vi "autonSample.vi"(0 "Auton Array":dbl[][](array[numeric]), 5 "MeasuredHeading":dbl, 9 "EncoderDistance":dbl) -> (4 "Left Drive":dbl(knob) scale=-1.0..1.0, 6 "Right Drive":dbl(knob) scale=-1.0..1.0, 10 "Turret Rotation":dbl, 14 "Feeder motor":dbl, 15 "Shooter motor output":dbl)   [LabVIEW 2011]
uses:
  Robot Global Data.vi
panel:
  in  "ShooterDesRate 2":dbl
  in  "ShooterEncRate 2":dbl
  in  "ShooterDesRate":dbl
  in  "ShooterEncRate":dbl
  in  "Balls Fired 2":i32
  in  "Balls Fired":i32
  out "Tzero":i64
  out "AccumDist":dbl
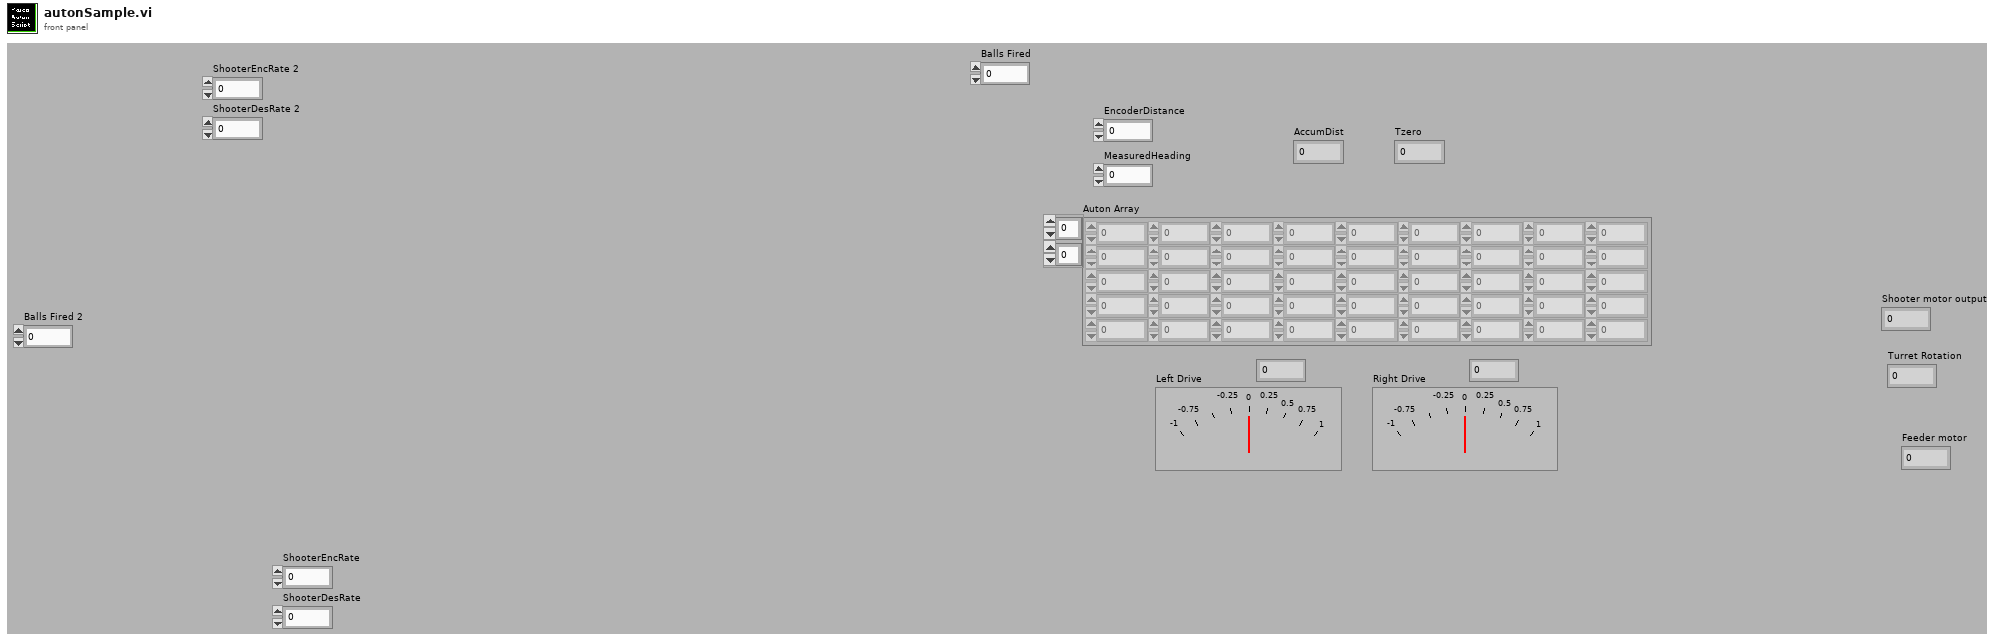
[diagram p1: front panel]
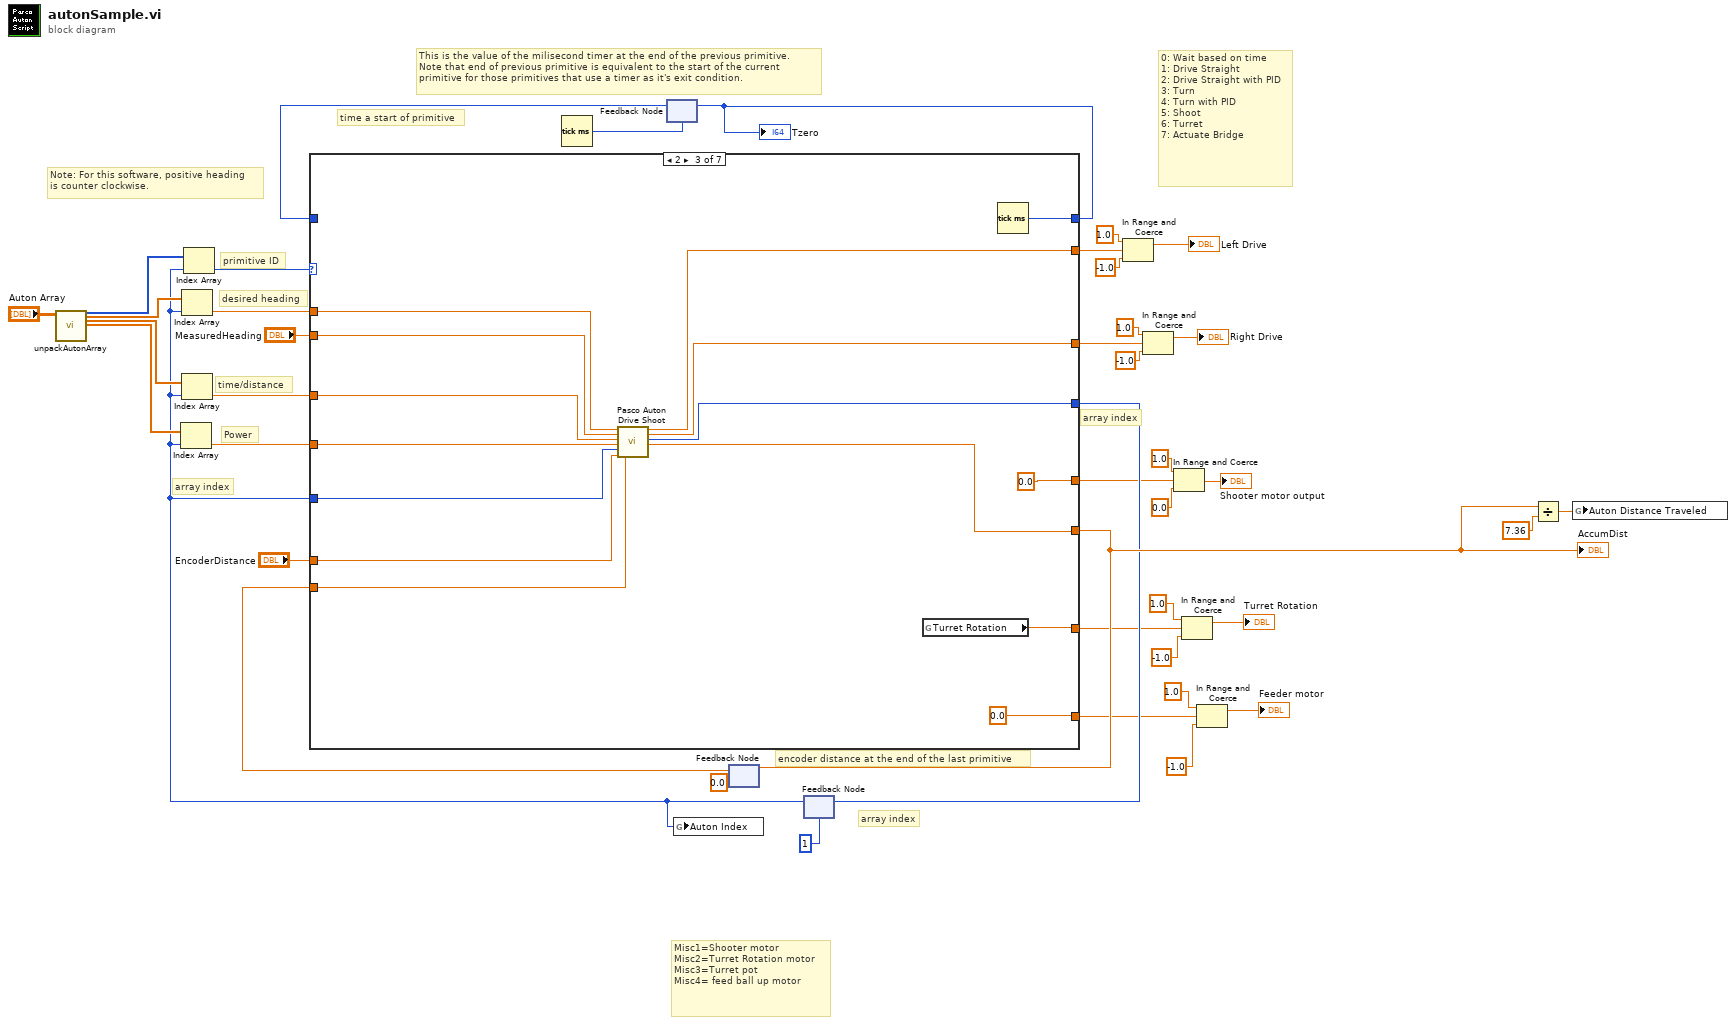
[diagram p0: block diagram]
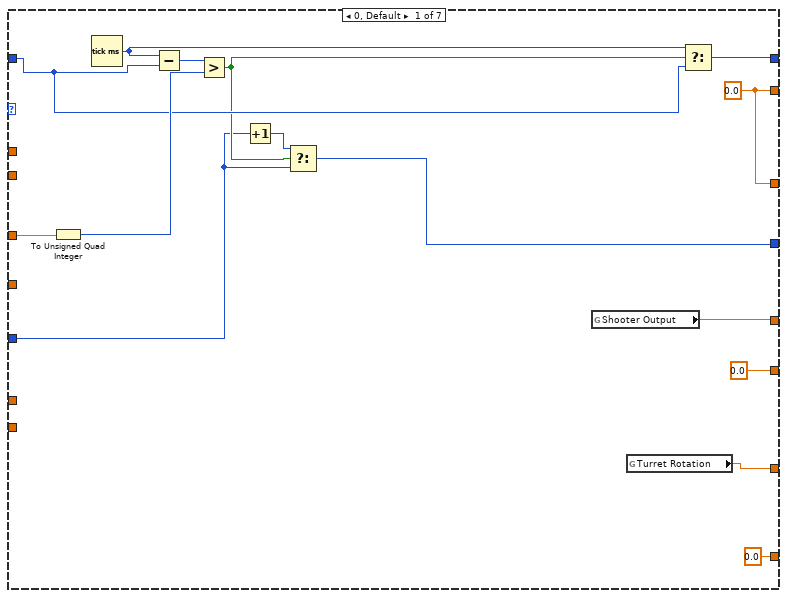
[diagram p2: hidden frame]
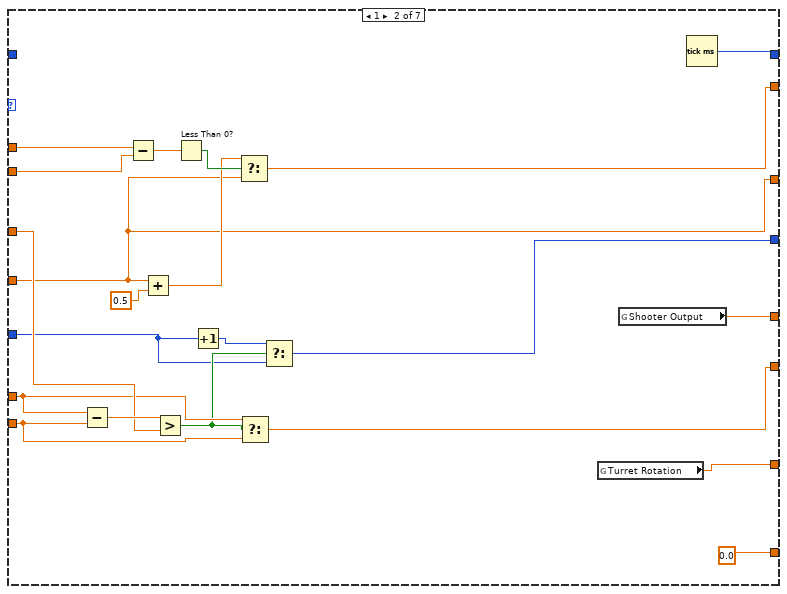
[diagram p3: hidden frame]
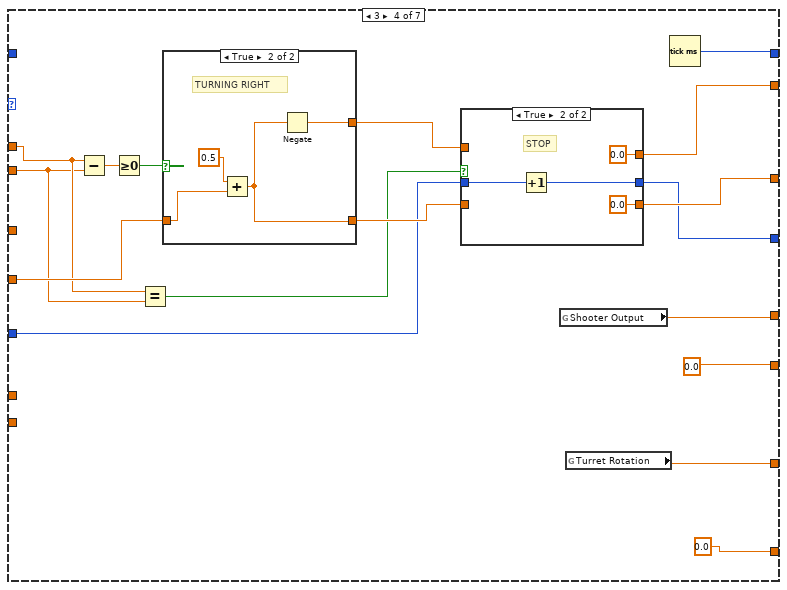
[diagram p4: hidden frame]
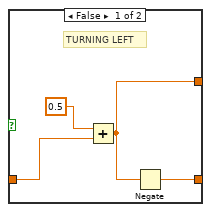
[diagram p6: hidden frame]
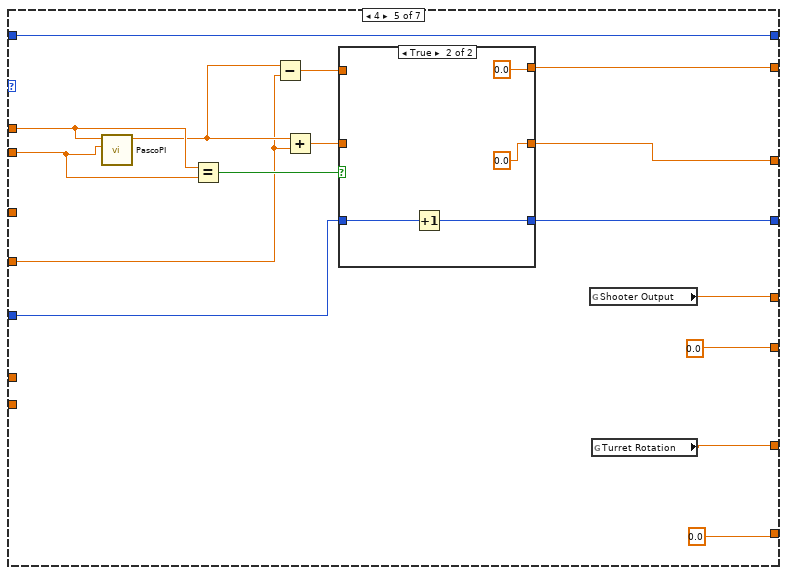
[diagram p7: hidden frame]
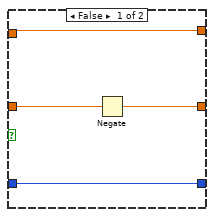
[diagram p8: hidden frame]
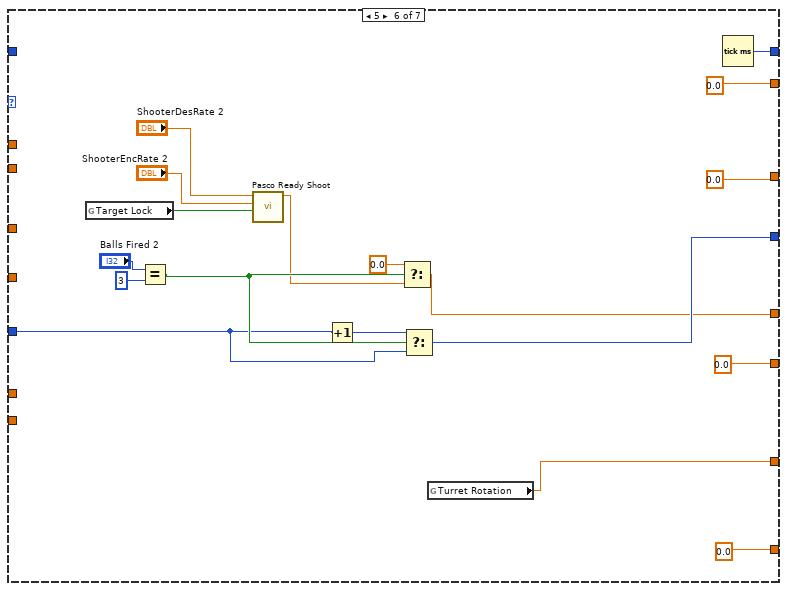
[diagram p9: hidden frame]
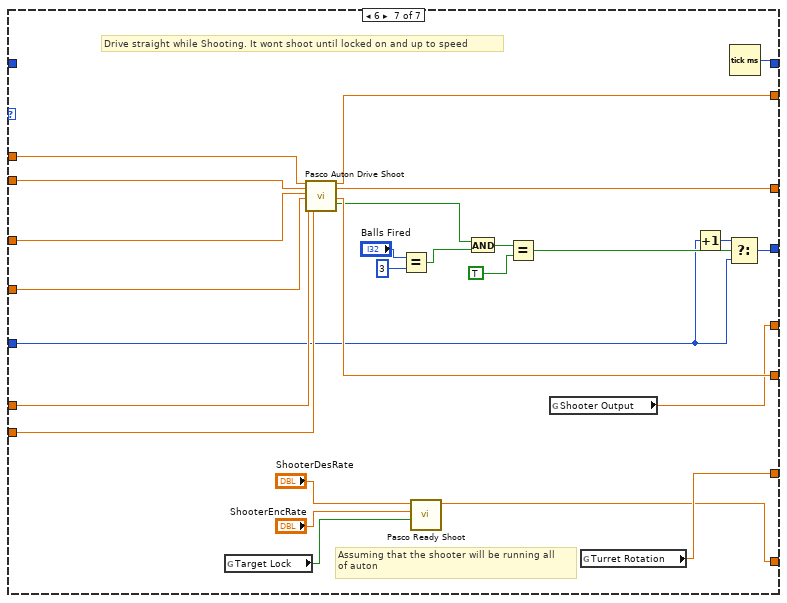
[diagram p10: hidden frame]
diagram:
  # "Misc1=Shooter motor\nMisc2=Turret Rotation motor\nMisc3=Turret pot\nMisc4= feed ball up motor"
  # "0: Wait based on time\n1: Drive Straight\n2: Drive Straight with PID\n3: Turn\n4: Turn with PID\n5: Shoot\n6: Turret\n7: Actuate Bridge"
  # "encoder distance at the end of the last primitive"
  # "Note: For this software, positive heading\nis counter clockwise."
  # "time a start of primitive"
  # "array index"
  # "array index"
  # "This is the value of the milisecond timer at the end of the previous primitive.\nNote that end of previous primitive is equivalent to the start of the current\nprimitive for those primitives that use a timer as it's exit condition."
  # "Power"
  # "array index"
  # "desired heading"
  # "primitive ID"
  # "time/distance"
  n1 = call "unpackAutonArray.vi"("all rows"="Auton Array") -> ("Primitive"=w41:i16[], "Heading"=w23:dbl[], "Distance/Time"=w24:dbl[], "Power"=w21:dbl[])  [unwired: 1 in, 22 out]
  n2 = Tick Count (ms)() -> (millisecond timer value=w35:u32)
  n3 = feedback #1(w35) -> (w39:u32)
  n4 = feedback #2(0.0 ("EncoderDistance")) -> (w20:dbl)
  n5 = feedback #3(1) -> (w2:i32)
  n6 = Index Array(array=w21, index=w2) -> (element=w37:dbl)
  n7 = Index Array(array=w23, index=w2) -> (element=w22:dbl)
  n8 = Index Array(array=w24, index=w2) -> (element=w38:dbl)
  n9 = Index Array(array=w41, index=w2) -> (element=w40:i16)
  n10 = case shown="2" w40 {
    tunnel: [w46 w63 w81 w99 w137 w161 w178] -> w15
    tunnel: w2 -> [w47 w64 w86 w98 w136 w154 w174]
    tunnel: [w57 w62 w92 w105 w141 w162 w172] -> w25
    tunnel: w39 -> [w53 _ _ _ w141 _ _]
    tunnel: w38 -> [w55 w71 w88 _ _ _ w191]
    tunnel: w22 -> [_ w77 w90 w107 w131 _ w193]
    tunnel: [w45 w73 w83 w101 w138 0.0 w187] -> w33
    tunnel: [w45 w59 w82 w104 w139 0.0 w186] -> w26
    tunnel: w37 -> [_ w59 w87 w109 w128 _ w190]
    tunnel: "EncoderDistance" -> [_ w70 w85 _ _ _ w189]
    tunnel: "MeasuredHeading" -> [_ w76 w89 w106 w132 _ w192]
    tunnel: [0.0 ("Encoder total") w67 w80 0.0 0.0 0.0 w185] -> w17
    tunnel: w20 -> [_ w69 w84 _ _ _ w188]
    tunnel: [w43 w58 0.0 ("Misc1  OUT") w94 w126 w160 w173] -> w11
    tunnel: [w44 w68 w79 w95 w127 w163 w176] -> w7
    tunnel: [0.0 ("Misc4 OUT") 0.0 0.0 0.0 0.0 0.0 w171] -> w3
    frame 0, Default {
      w45 = 0.0 ("Numeric")
      n11 = To Unsigned Quad Integer(1:w55) -> (0:w54:u64)
      n12 = Tick Count (ms)() -> (millisecond timer value=w52:u32)
      n13 = Subtract(x=w52, y=w53) -> (x-y=w56:u32)
      n14 = Greater?(x=w56, y=w54) -> (0:w49:bool)
      n15 = Increment(x=w47) -> (x+1=w48:i32)
      n16 = Select(t=w48, s=w49, f=w47) -> (s? t:f=w46:i32)
      n17 = global read "Robot Global Data.vi" "Shooter Output"() -> (w43:dbl)
      n18 = global read "Robot Global Data.vi" "Turret Rotation"() -> (w44:dbl)
      n19 = Select(t=w52, s=w49, f=w53) -> (s? t:f=w57:u32)
    }
    frame 1 {
      n20 = Subtract(x=w70, y=w69) -> (x-y=w72:dbl)
      n21 = Subtract(x=w77, y=w76) -> (x-y=w61:dbl)
      n22 = Add(x=w59, y=0.5) -> (x+y=w60:dbl)
      n23 = Greater?(x=w72, y=w71) -> (0:w66:bool)
      n24 = Less Than 0?(x=w61) -> (x < 0?=w75:bool)
      n25 = Increment(x=w64) -> (x+1=w65:i32)
      n26 = Select(t=w60, s=w75, f=w59) -> (s? t:f=w73:dbl)
      n27 = Select(t=w70, s=w66, f=w69) -> (s? t:f=w67:dbl)
      n28 = Select(t=w65, s=w66, f=w64) -> (s? t:f=w63:i32)
      n29 = global read "Robot Global Data.vi" "Turret Rotation"() -> (w68:dbl)
      n30 = global read "Robot Global Data.vi" "Shooter Output"() -> (w58:dbl)
      n31 = Tick Count (ms)() -> (millisecond timer value=w62:u32)
    }
    frame 2 {
      n32 = call "Pasco Auton Drive Shoot.vi"("Desired Heading"=w90, "Actual Heading"=w89, "time/distance"=w88, "Power"=w87, "Array"=w86, "Encoder total"=w85, "Encoder Return"=w84) -> ("Left Drive"=w83:dbl, "Right Drive"=w82:dbl, "Array Out"=w81:i32, "Encoder total"=w80:dbl)  [unwired: 8 in, 1 out]
      n33 = global read "Robot Global Data.vi" "Turret Rotation"() -> (w79:dbl)
      n34 = Tick Count (ms)() -> (millisecond timer value=w92:u32)
    }
    frame 3 {
      n35 = Subtract(x=w107, y=w106) -> (x-y=w110:dbl)
      n36 = Greater Or Equal To 0?(x=w110) -> (x >= 0?=w108:bool)
      n37 = Equal?(x=w107, y=w106) -> (x = y?=w100:bool)
      n38 = case shown="True" w108 {
        tunnel: w109 -> [w120 w122]
        tunnel: [w118 w124] -> w102
        tunnel: [w119 w123] -> w103
        frame False {
          # "TURNING LEFT"
          n39 = Add(x=0.5, y=w120) -> (x+y=w118:dbl)
          n40 = Negate(x=w118) -> (-x=w119:dbl)
        }
        frame True {
          # "TURNING RIGHT"
          n41 = Add(x=0.5, y=w122) -> (x+y=w123:dbl)
          n42 = Negate(x=w123) -> (-x=w124:dbl)
        }
      }
      n43 = case shown="True" w100 {
        tunnel: w98 -> [w113 w117]
        tunnel: [w113 w116] -> w99
        tunnel: [w112 0.0] -> w104
        tunnel: w103 -> [w112 _]
        tunnel: [w111 0.0] -> w101
        tunnel: w102 -> [w111 _]
        frame False {
          # "DRIVE"
        }
        frame True {
          # "STOP"
          n44 = Increment(x=w117) -> (x+1=w116:i32)
        }
      }
      n45 = global read "Robot Global Data.vi" "Shooter Output"() -> (w94:dbl)
      n46 = global read "Robot Global Data.vi" "Turret Rotation"() -> (w95:dbl)
      n47 = Tick Count (ms)() -> (millisecond timer value=w105:u32)
    }
    frame 4 {
      n48 = call "PascoPI.vi"("Feedback"=w132, "Setpoint"=w131) -> ("Motor Output"=w130:dbl)  [unwired: 9 in]
      n49 = Equal?(x=w131, y=w132) -> (x = y?=w134:bool)
      n50 = Subtract(x=w130, y=w128) -> (x-y=w133:dbl)
      n51 = Add(x=w130, y=w128) -> (x+y=w129:dbl)
      n52 = case shown="True" w134 {
        tunnel: w133 -> [w143 _]
        tunnel: [w145 0.0] -> w139
        tunnel: [w143 0.0] -> w138
        tunnel: [w144 w148] -> w137
        tunnel: w136 -> [w144 w149]
        tunnel: w129 -> [w142 _]
        frame False {
          n53 = Negate(x=w142) -> (-x=w145:dbl)
        }
        frame True {
          n54 = Increment(x=w149) -> (x+1=w148:i32)
        }
      }
      n55 = global read "Robot Global Data.vi" "Shooter Output"() -> (w126:dbl)
      n56 = global read "Robot Global Data.vi" "Turret Rotation"() -> (w127:dbl)
    }
    frame 5 {
      n57 = global read "Robot Global Data.vi" "Target Lock"() -> (w153:bool)
      n58 = Equal?(x="Balls Fired 2", y=3) -> (x = y?=w157:bool)
      n59 = call "Pasco Ready Shoot.vi"("Light On/Locked On"=w153, "ShooterEncRate"="ShooterEncRate 2", "ShooterDesRate"="ShooterDesRate 2") -> ("Feeder Output"=w150:dbl)  [unwired: 8 in]
      n60 = Increment(x=w154) -> (x+1=w155:i32)
      n61 = Select(t=0.0, s=w157, f=w150) -> (s? t:f=w160:dbl)
      n62 = Select(t=w155, s=w157, f=w154) -> (s? t:f=w161:i32)
      n63 = global read "Robot Global Data.vi" "Turret Rotation"() -> (w163:dbl)
      n64 = Tick Count (ms)() -> (millisecond timer value=w162:u32)
    }
    frame 6 {
      # "Drive straight while Shooting. It wont shoot until locked on and up to speed"
      # "Assuming that the shooter will be running all\nof auton"
      n65 = global read "Robot Global Data.vi" "Target Lock"() -> (w168:bool)
      n66 = call "Pasco Auton Drive Shoot.vi"("Desired Heading"=w193, "Actual Heading"=w192, "time/distance"=w191, "Power"=w190, "Encoder total"=w189, "Encoder Return"=w188) -> ("Left Drive"=w187:dbl, "Right Drive"=w186:dbl, "Encoder total"=w185:dbl, "Complete?"=w184:bool)  [unwired: 9 in, 1 out]
      n67 = Equal?(x="Balls Fired", y=3) -> (x = y?=w183:bool)
      n68 = call "Pasco Ready Shoot.vi"("Light On/Locked On"=w168, "ShooterEncRate"="ShooterEncRate", "ShooterDesRate"="ShooterDesRate") -> ("Feeder Output"=w171:dbl)  [unwired: 8 in]
      n69 = And(x=w184, y=w183) -> (x .and. y?=w180:bool)
      n70 = Equal?(x=w180, y=TRUE) -> (x = y?=w175:bool)
      n71 = global read "Robot Global Data.vi" "Shooter Output"() -> (w173:dbl)
      n72 = global read "Robot Global Data.vi" "Turret Rotation"() -> (w176:dbl)
      n73 = Increment(x=w174) -> (x+1=w177:i32)
      n74 = Select(t=w177, s=w175, f=w174) -> (s? t:f=w178:i32)
      n75 = Tick Count (ms)() -> (millisecond timer value=w172:u32)
    }
  }
  "AccumDist" <- w17
  "Tzero" <- w25
  n76 = feedback-in #1(w25) -> ()
  n77 = global write "Robot Global Data.vi" "Auton Index"(w2) -> ()
  n78 = feedback-in #2(w17) -> ()
  n79 = feedback-in #3(w15) -> ()
  n80 = In Range and Coerce(upper limit=1.0, x=w33, lower limit=-1.0) -> (coerced(x)=→"Left Drive":dbl)  [unwired: 1 out]
  n81 = In Range and Coerce(upper limit=1.0, x=w26, lower limit=-1.0) -> (coerced(x)=→"Right Drive":dbl)  [unwired: 1 out]
  n82 = In Range and Coerce(upper limit=1.0, x=w11, lower limit=0.0) -> (coerced(x)=→"Shooter motor output":dbl)  [unwired: 1 out]
  n83 = In Range and Coerce(upper limit=1.0, x=w7, lower limit=-1.0) -> (coerced(x)=→"Turret Rotation":dbl)  [unwired: 1 out]
  n84 = In Range and Coerce(upper limit=1.0, x=w3, lower limit=-1.0) -> (coerced(x)=→"Feeder motor":dbl)  [unwired: 1 out]
  n85 = Divide(x=w17, y=7.36) -> (x/y=w1:dbl)
  n86 = global write "Robot Global Data.vi" "Auton Distance Traveled"(w1) -> ()
